vi "GUNSC_LibGetFPA.vi"(7 "Extensions":u16[](array[numeric]), 8 "error in (no error)":errorcluster, 10 "readmode":string, 11 "detext":bool) -> (0 "error out":errorcluster, 2 "num amplifiers":i32, 3 "Extensions_out":u16[](array[numeric]), 4 "totysize":i32, 6 "totxsize":i32)   [LabVIEW 2016]
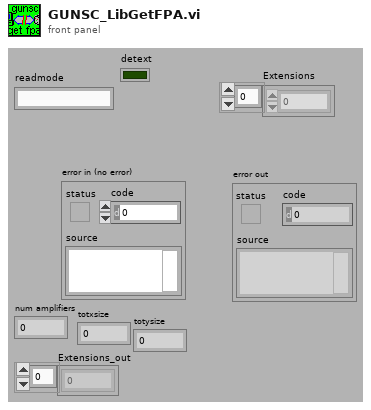
[diagram p1: front panel]
types:
  T1 = typedef "GEOM_CorrectedFPA.ctl" = cluster{"readmode":string, "amplifiers":cluster{"number":i32, "xstart":i32, "ystart":i32}[], "totxsize":i32, "totysize":i32, "maxxdim":i32, "maxydim":i32, "numxamps":i32, "numyamps":i32, "totxdata":i32, "totydata":i32, "xdataamp":i32, "ydataamp":i32, "totpixels":i32}
  T2 = typedef "GEOM_Amplifier.ctl" = cluster{"number":i32, "type":T3, "rotated":i16, "fliped":u16, "FPAcoord":cluster{"xstart":i32, "ystart":i32}, "Physical_size":cluster{"columns":i32, "rows":i32}, "predata":cluster{"columns":i32, "rows":i32}, "postdata":cluster{"columns":i32, "rows":i32}, "Req ROIs":T4, "Corr ROI":T4, "Detnumber":i32, "ampID":string, "discard":i32}
  T3 = typedef "GEOM_AmpType.ctl" = u16
  T4 = typedef "GEOM_ROI.ctl" = T5[]
  T5 = typedef "GEOM_Coords.ctl" = cluster{"xstart":u32, "ystart":u32, "xsize":u32, "ysize":u32}
  T6 = typedef "GEOM_DetSummaryStruct.ctl" = cluster{"detxpos":i32, "detypos":i32, "cols":i32, "rows":i32, "nxamps":i32, "nyamps":i32, "number":i32, "discard":i32, "totcols":i32, "totrows":i32, "readmode":string}
  T7 = cluster{"number":i32, "xstart":i32, "ystart":i32}[]
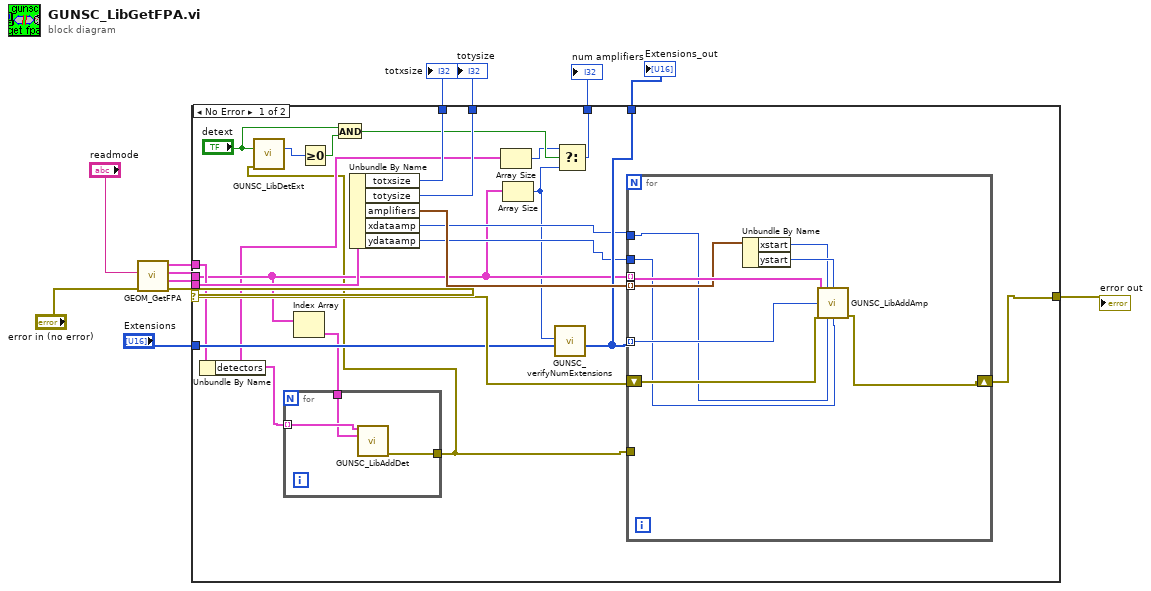
[diagram p0: block diagram]
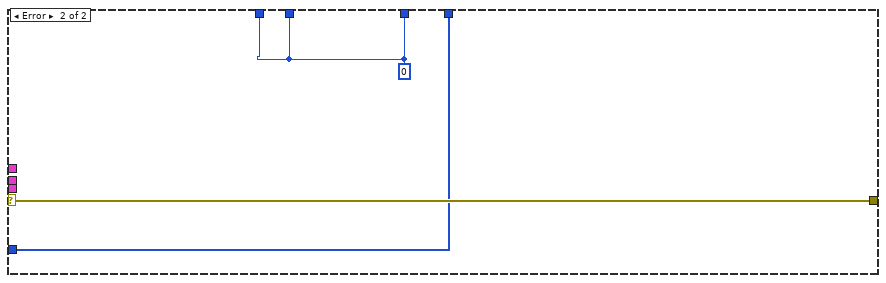
[diagram p2: hidden frame]
diagram:
  n1 = call "GEOM_GetFPA.vi"("error in (no error)"="error in (no error)", "readmode"="readmode") -> ("error out"=w10:errorcluster, "CorrectedFPACoord"=w6:T1, "amplifiers"=w11:T2[], "detreadmodes"=w1:cluster{"name":string, "detectors":T6[]})  [unwired: 1 in, 5 out]
  n2 = case shown="No Error" w10 {
    selector: w10 -> [w34 w49]
    tunnel: w11 -> [w20 _]
    tunnel: [w33 w49] -> w9
    tunnel: [w14 w48] -> w7
    tunnel: w6 -> [w32 _]
    tunnel: [w28 w48] -> w5
    tunnel: [w27 w48] -> w4
    tunnel: "Extensions" -> [w30 w47]
    tunnel: [w29 w47] -> w2
    tunnel: w1 -> [w21 _]
    frame No Error {
      n3 = Unbundle By Name(w21) -> ("detectors"=w18:T6[])
      n4 = Index Array(array=w20) -> (element=w19:T2)  [unwired: 1 in]
      n5 = for {
        tunnel: w18 -> [w37] mode=indexing
        tunnel: w19 -> [w36]
        tunnel: [w35] -> w13
        n6 = call "GUNSC_LibAddDet.vi"("detector"=w37, "Amplifier"=w36) -> ("error out"=w35:errorcluster)  [unwired: 1 in, 12 out]
      }
      n7 = call "GUNSC_LibDetExt.vi"("detext"="detext", "error in (no error)"=w13) -> ("return value"=w24:i32)  [unwired: 13 out]
      n8 = Greater Or Equal To 0?(x=w24) -> (x >= 0?=w23:bool)
      n9 = And(x="detext", y=w23) -> (x .and. y?=w17:bool)
      n10 = Unbundle By Name(w32) -> ("totxsize"=w28:i32, "totysize"=w27:i32, "amplifiers"=w31:T7, "xdataamp"=w26:i32, "ydataamp"=w25:i32)
      n11 = Array Size(array=w18) -> (size(s)=w16:i32)
      n12 = Array Size(array=w20) -> (size(s)=w15:i32)
      n13 = call "GUNSC_verifyNumExtensions.vi"("current_extensions"=w30, "geom_num_amplif"=w15) -> ("current_extensions out"=w29:u16[])  [unwired: 8 out]
      n14 = Select(t=w16, s=w17, f=w15) -> (s? t:f=w14:i32)
      n15 = for {
        tunnel: w20 -> [w44] mode=indexing
        shift-right: [w45] -> w33
        shift-left: w34 -> [w46]
        tunnel: w31 -> [w43] mode=indexing
        tunnel: w29 -> [w40] mode=indexing
        tunnel: w26 -> [w39]
        tunnel: w25 -> [w38]
        tunnel: w13 -> [_]
        n16 = Unbundle By Name(w43) -> ("xstart"=w41:i32, "ystart"=w42:i32)
        n17 = call "GUNSC_LibAddAmp.vi"("correctedxstart"=w41, "correctedystart"=w42, "Amplifier"=w44, "extension"=w40, "error in (no error)"=w46, "xdata"=w39, "ydata"=w38) -> ("error out"=w45:errorcluster)  [unwired: 3 in, 5 out]
      }
    }
    frame Error {
      w48 = 0
    }
  }
  "error out" <- w9
  "num amplifiers" <- w7
  "totxsize" <- w5
  "totysize" <- w4
  "Extensions_out" <- w2
